vi "XML Load XML.vi"(8 "Error In":errorcluster, 11 "path to XML document in":path) -> (0 "Error Out":errorcluster, 3 "Refnum out":refnum<k20>)   [LabVIEW 2014]
uses:
  <vilib>/xml/NI_XML.lvlib
  <resource>/objmgr/DOMUserDefRef.rc
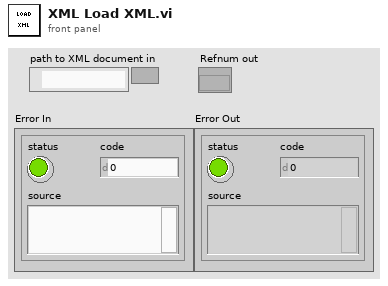
[diagram p1: front panel]
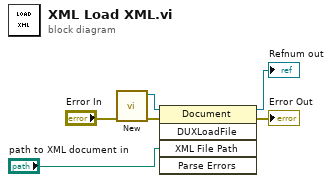
[diagram p0: block diagram]
diagram:
  n1 = call <vilib>:"New.vi"("error in (no error)"="Error In") -> ("error out"=w2:errorcluster, "DOM document out"=w5:refnum<k20>)  [unwired: 7 in]
  n2 = invoke class="Document" method="DUXLoadFile"(reference=w5, error in=w2, "XML File Path"="path to XML document in") -> (reference out=→"Refnum out":refnum<k20>, error out=→"Error Out":errorcluster)  [unwired: 2 in, 3 out]
